vi "Initialize Amplitudes.vi"(0 "MRN in":refnum<class "Moving Ripple Noise.lvclass">, 7 "Level in":refnum<class "Level.lvclass">, 11 "error in (no error)":errorcluster) -> (4 "MRN out":refnum<class "Moving Ripple Noise.lvclass">, 15 "error out":errorcluster)   [LabVIEW 2020, in "Moving Ripple Noise.lvclass"]
uses:
  Moving Ripple Noise.lvclass
  Level/Level.lvclass
  Moving Ripple Noise.lvclass/Moving Ripple Noise.ctl
  Level/Level.lvclass/Level.ctl
  c1d9fe8f-1f84-4bea-ab25-480226708dd3.vi
  6bf28cdf-27f1-4c06-b314-ce1e8a5d1a8a.vi
  Level/Read Units.vi
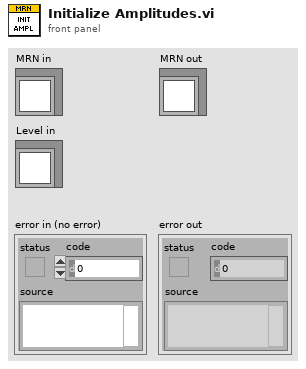
[diagram p1: front panel]
types:
  T1 = typedef "Level.lvclass/LevelUnits.ctl" = enum16{"dB atten", "dB SPL", "dB Vrms", "Volts", "dB mW", "mW", "dB HL", "dB SL"}
  T2 = cluster{"Freq (Hz)":dbl[], "Mag (dB SPL)":dbl[], "Phase (deg)":dbl[]}
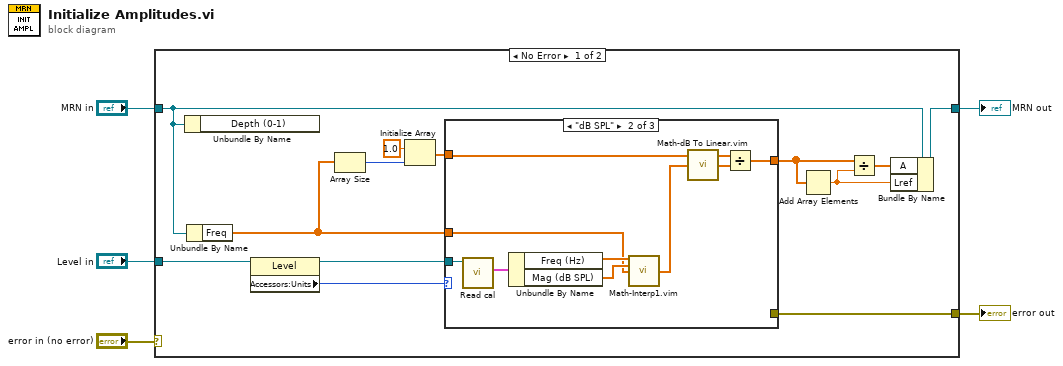
[diagram p0: block diagram]
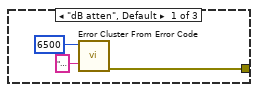
[diagram p2: hidden frame]
diagram:
  n1 = case shown="No Error" "error in (no error)" {
    selector: "error in (no error)" -> [_ w33]
    tunnel: [w12 w33] -> w4
    tunnel: [w13 w32] -> w2
    tunnel: "MRN in" -> [w10 w32]
    tunnel: "Level in" -> [w18 _]
    frame No Error {
      n2 = Unbundle By Name(w10) -> ()  [unwired: 1 out]
      n3 = Unbundle By Name(w10) -> ("Freq"=w15:dbl[])
      n4 = property class="Level"(reference=w18) -> (reference out=w17:refnum<class "Level.lvclass">, "Accessors:Units"=w16:T1)  [unwired: 1 in, 1 out]
      n5 = Array Size(array=w15) -> (size(s)=w11:i32)
      n6 = Initialize Array(1.0 ("element"), w11) -> (w14:dbl[])
      n7 = case shown="\"dB SPL\"" w16 {
        tunnel: w17 -> [_ w29 _]
        tunnel: [w19 _ _] -> w12
        tunnel: w15 -> [_ w22 _]
        tunnel: w14 -> [_ w26 w31]
        tunnel: [_ w25 w31] -> w8
        frame "dB atten", Default {
          n8 = call <vilib>:"Error Cluster From Error Code.vi"("error message (\"\")"="Moving Ripple Noise level must be in units of dB SPL or dB Vrms" ("error message (\"\")"), "error code (0)"=6500) -> ("error out"=w19:errorcluster)  [unwired: 7 in]
        }
        frame "dB SPL" {
          n9 = call "Read cal.vi"("Level in"=w29) -> ("cal"=w30:T2)  [unwired: 8 in, 2 out]
          n10 = Unbundle By Name(w30) -> ("Freq (Hz)"=w28:dbl[], "Mag (dB SPL)"=w27:dbl[])
          n11 = call "Math-Interp1.vim"("X"=w28, "Y"=w27, "U"=w22) -> ("V"=w24:dbl[])  [unwired: 12 in]
          n12 = call "Math-dB To Linear.vim"("dB"=w24) -> ("linear"=w23:dbl[])
          n13 = Divide(x=w26, y=w23) -> (x/y=w25:dbl[])
        }
        frame "dB Vrms" {
        }
      }
      n14 = Add Array Elements(numeric array=w8) -> (sum=w6:dbl)
      n15 = Divide(x=w8, y=w6) -> (x/y=w7:dbl[])
      n16 = Bundle By Name(cluster=w10, "A"=w7, "Lref"=w6) -> (w13:refnum<class "Moving Ripple Noise.lvclass">)
    }
    frame Error {
    }
  }
  "error out" <- w4
  "MRN out" <- w2
